vi "Match Multiple Pattern.vi"(7 "delimiter (|)":string="|", 8 "offset (0)":i32, 10 "regular expression":string, 11 "string":string) -> (0 "Found?":bool, 1 "after substring":string, 2 "match substring":string, 3 "before substring":string, 4 "pattern matched":string)   [LabVIEW 2017]
doc: "Searches string for the first of several regular expressions, beginning at offset. The expressions are listed in regular expression separated by delimiter, and the outputs split string into the before, match, pattern matched and after substrings."
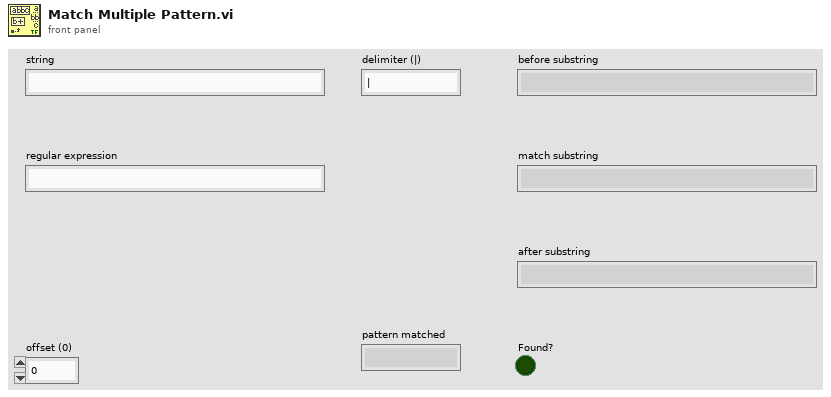
[diagram p1: front panel]
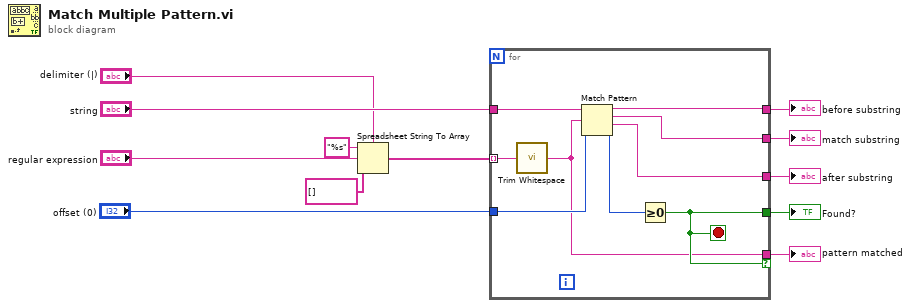
[diagram p0: block diagram]
diagram:
  n1 = Spreadsheet String To Array(delimiter (Tab)="delimiter (|)", format string="%s", spreadsheet string="regular expression", array type (2D Dbl)=string[] [] ("Array of Strings")) -> (array=w4:string[])
  n2 = for {
    tunnel: "offset (0)" -> [w20]
    tunnel: [w17] -> w8
    tunnel: [w14] -> w7
    tunnel: "string" -> [w21]
    tunnel: [w19] -> w10
    tunnel: w4 -> [w15] mode=indexing
    tunnel: [w18] -> w9
    tunnel: [w13] -> w3 if=w14
    stop <- w14 stop-if-true
    n3 = call <vilib>:"Trim Whitespace.vi"("string"=w15) -> ("trimmed string"=w13:string)  [unwired: 1 in]
    n4 = Match Pattern(string=w21, regular expression=w13, offset (0)=w20) -> (before substring=w19:string, match substring=w18:string, after substring=w17:string, offset past match=w16:i32)
    n5 = Greater Or Equal To 0?(x=w16) -> (x >= 0?=w14:bool)
  }
  "before substring" <- w10
  "match substring" <- w9
  "after substring" <- w8
  "Found?" <- w7
  "pattern matched" <- w3
